vi "ERR HANDLER - Log Error.vi"(8 "error":errorcluster) -> (0 "error out":errorcluster)   [LabVIEW 2013]
uses:
  <vilib>/Utility/error.llb/DialogType.ctl
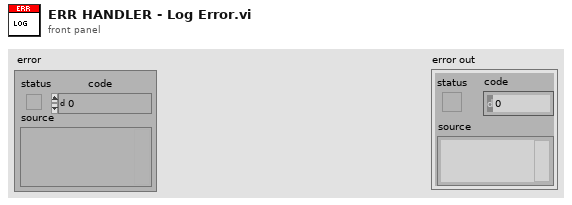
[diagram p1: front panel]
types:
  T1 = typedef "DialogType.ctl" = u16
  T2 = enum16{"open", "replace", "create", "open or create", "replace or create", "replace or create with confirmation"}
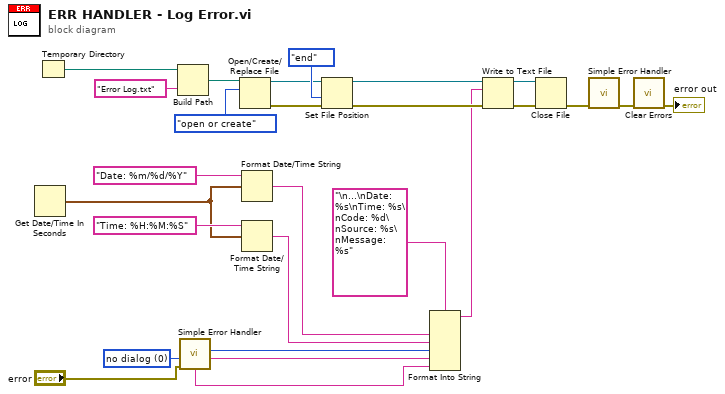
[diagram p0: block diagram]
diagram:
  w6 = T1 0 items=["no dialog", "OK message", "continue or stop message", "OK message + warnings", "continue/stop + warnings"] ("type of dialog (OK msg:1)")
  n1 = Get Date/Time In Seconds() -> (seconds since 1Jan1904=w7:timestamp)
  n2 = Temporary Directory() -> (w1:path)
  n3 = Build Path(base path=w1, name or relative path="Error Log.txt") -> (appended path=w24:path)
  n4 = call <vilib>:"Simple Error Handler.vi"("type of dialog (OK msg:1)"=w6, "error in (no error)"="error") -> ("code out"=w2:i32, "source out"=w3:string, "message"=w4:string)  [unwired: 3 in, 2 out]
  n5 = Open/Create/Replace File(file path (use dialog)=w24, operation (0:open)=T2."open or create") -> (refnum out=w12:refnum<file>, error out=w10:errorcluster)  [unwired: 4 in, 1 out]
  n6 = Format Date/Time String(time format string (%c)="Date: %m/%d/%Y", seconds (now)=w7) -> (date/time string=w17:string)  [unwired: 1 out]
  n7 = Format Date/Time String(time format string (%c)="Time: %H:%M:%S", seconds (now)=w7) -> (date/time string=w16:string)  [unwired: 1 out]
  n8 = Set File Position(refnum=w12, from (0:start)=enum16{"start", "end", "current"}."end", error in=w10) -> (refnum out=w11:refnum<file>, error out=w9:errorcluster)  [unwired: 1 in]
  n9 = Format Into String(format string="\n...\nDate: %s\nTime: %s\nCode: %d\nSource: %s\nMessage: %s", w17, w16, w2, w3, w4) -> (resulting string=w8:string)  [unwired: 2 in, 1 out]
  n10 = Write to Text File(file (use dialog)=w11, text=w8, error in=w9) -> (refnum out=w22:refnum<file>, error out=w23:errorcluster)  [unwired: 1 in, 1 out]
  n11 = Close File(refnum=w22, error in=w23) -> (error out=w21:errorcluster)  [unwired: 1 out]
  n12 = call <vilib>:"Simple Error Handler.vi"("error in (no error)"=w21) -> ("error out"=w15:errorcluster)  [unwired: 4 in, 4 out]
  n13 = call <vilib>:"Clear Errors.vi"("error in (no error)"=w15) -> ("error out"=→"error out":errorcluster)  [unwired: 6 in]
